vi "Destroy Q.vi"(7 "Q Ref In":refnum<queue>, 8 "error in":errorcluster) -> (0 "error out":errorcluster, 3 "Flushed Elements":T1[](array[typedef]))   [LabVIEW 2025, in "Q Wrappers.lvlib"]
uses:
  Q Wrappers.lvlib
  Q Packet.ctl
panel:
  in  "Force Destory (T)":bool=TRUE
  out "Queue ID":string
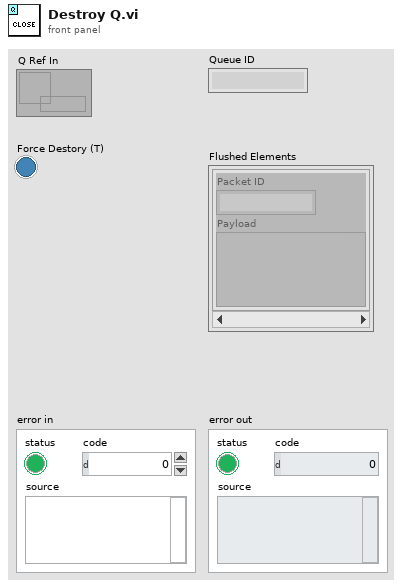
[diagram p1: front panel]
types:
  T1 = typedef "Q Packet.ctl" = cluster{"Packet ID":string, "Payload":variant}
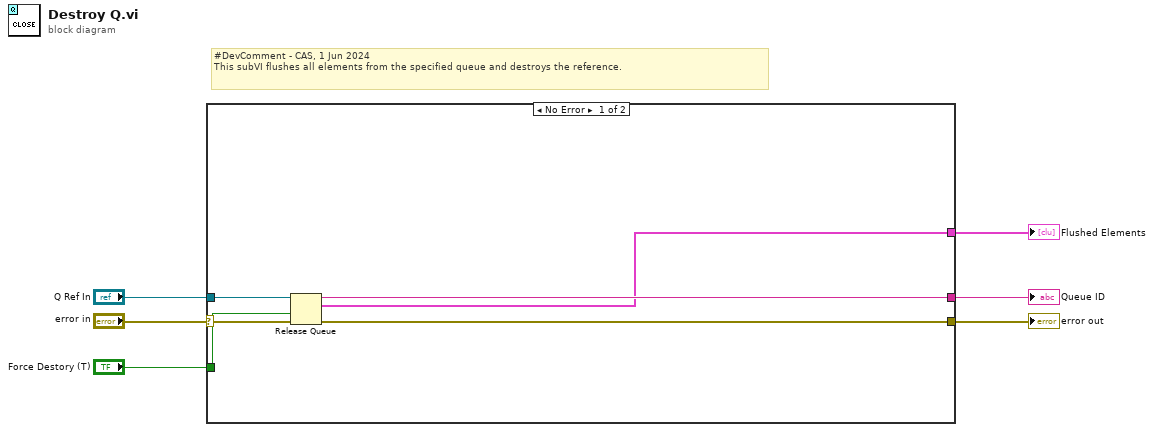
[diagram p0: block diagram]
diagram:
  # "#DevComment - CAS, 1 Jun 2024\nThis subVI flushes all elements from the specified queue and destroys the reference."
  n1 = case shown="No Error" "error in" {
    selector: "error in" -> [w9 w13]
    tunnel: [w12 w13] -> w5
    tunnel: [w11 _] -> w2
    tunnel: "Q Ref In" -> [w10 _]
    tunnel: [w8 _] -> w3
    tunnel: "Force Destory (T)" -> [w7 _]
    frame No Error {
      n2 = Release Queue(queue=w10, force destroy? (F)=w7, error in (no error)=w9) -> (queue name=w11:string, remaining elements=w8:T1[], error out=w12:errorcluster)
    }
    frame Error {
    }
  }
  "error out" <- w5
  "Flushed Elements" <- w3
  "Queue ID" <- w2
